vi "Set Drive Speed.vi"(10 "Speed":dbl, 11 "Execute?":bool) -> (3 "Done":bool)   [LabVIEW 2012]
uses:
  Globals/Useful Values.vi
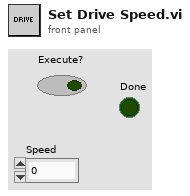
[diagram p1: front panel]
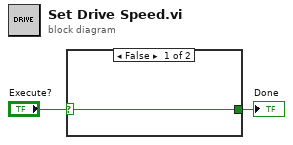
[diagram p0: block diagram]
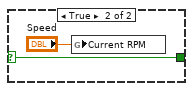
[diagram p2: hidden frame]
diagram:
  n1 = case shown="False" "Execute?" {
    selector: "Execute?" -> [w3 w4]
    tunnel: [w3 w4] -> w1
    frame False {
    }
    frame True {
      n2 = global write "Useful Values.vi" "Current RPM"("Speed") -> ()
    }
  }
  "Done" <- w1
